vi "Alarm Voice.vi"(2 "Volume Control":i32(knob)=75 min=0 max=100 step=1 scale=0.0..100.0, 3 "Speech Rate":i32(knob) min=-10 max=10 step=1 scale=-10.0..10.0, 4 "String":string="  F  I  C  A  -  7  8  4  1  Hi Alarm 中         故障發生") -> (1 "Voice error":errorcluster)   [LabVIEW 2018]
panel:
  in  "Menu Ring":u16(ring) items=["Microsoft Hanhan Desktop - Chinese (Taiwan)", "Microsoft Zira Desktop - English (United States)", "Microsoft David Desktop - English (United States)"]
  in  "SpeechLib.ISpeechVoice (In)":refnum<k7>
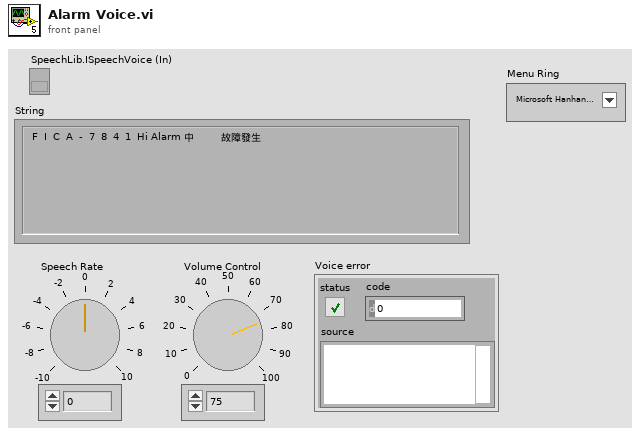
[diagram p1: front panel]
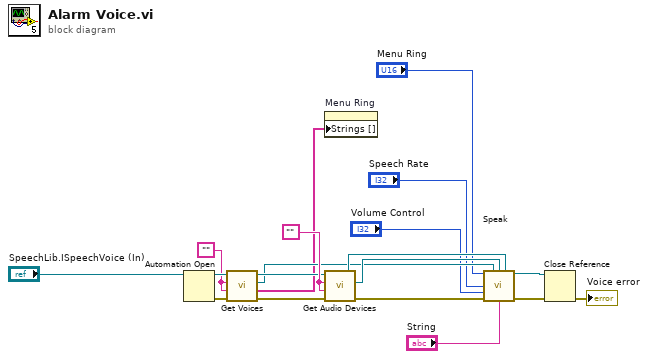
[diagram p0: block diagram]
diagram:
  w16 = ""
  w17 = ""
  n1 = Automation Open(Automation Refnum="SpeechLib.ISpeechVoice (In)") -> (Automation Refnum=w18:refnum<k7>, error out=w7:errorcluster)  [unwired: 3 in]
  n2 = call "Get Voices.vi"("error out"=w7, "OptionalAttributes"=w17, "RequiredAttributes"=w17, "SpeechLib.ISpeechVoice (In)"=w18) -> ("error in (no error)"=w6:errorcluster, "Voice Names"=w1:string[], "GetVoices"=w12:refnum<k7>, "SpeechLib.ISpeechVoice (Out)"=w15:refnum<k7>)
  n3 = property on="Menu Ring" class="Ring (strict)"("Strings []"=w1) -> ()  [unwired: 2 in, 2 out]
  n4 = call "Get Audio Devices.vi"("error out"=w6, "OptionalAttributes"=w16, "RequiredAttributes"=w16, "SpeechLib.ISpeechVoice (In)"=w15) -> ("error in (no error)"=w5:errorcluster, "GetAudioOutputs"=w13:refnum<k7>, "SpeechLib.ISpeechVoice (Out)"=w14:refnum<k7>)  [unwired: 1 out]
  n5 = call "Speak.vi"("voice"="Menu Ring", "GetVoices"=w12, "GetAudioOutputs"=w13, "SpeechLib.ISpeechVoice (In)"=w14, "Speech Rate"="Speech Rate", "Volume Control"="Volume Control", "error in"=w5, "String"="String") -> ("SpeechLib.ISpeechVoice (Out)"=w11:refnum<k7>, "error out (no error)"=w4:errorcluster)  [unwired: 4 in, 2 out]
  n6 = Close Reference(reference=w11, error in (no error)=w4) -> (error out=→"Voice error":errorcluster)
